vi "StopCalibration.vi"(7 "LVWSR":refnum<class "Web Request.lvclass">) -> ()   [LabVIEW 2014]
uses:
  <vilib>/wsapi/Web Request.lvclass
  Controller/Messages/Send Stop Calibration MSG/Send Stop Calibration MSG.lvclass
  Controller/Controller.lvclass
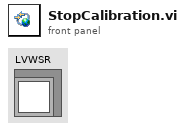
[diagram p1: front panel]
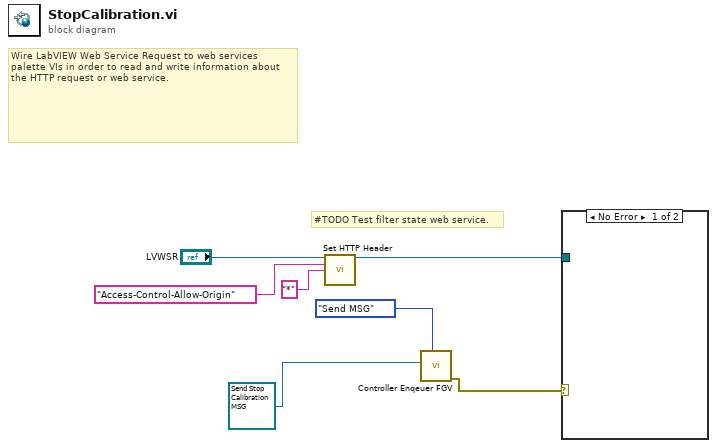
[diagram p0: block diagram]
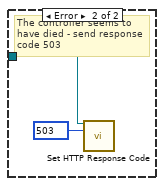
[diagram p2: hidden frame]
diagram:
  # "#TODO Test filter state web service."
  # "Wire LabVIEW Web Service Request to web services palette VIs in order to read and write information about the HTTP request or web service."
  n1 = call <vilib>:"Set HTTP Header.vi"("LabVIEW Web Service Request"="LVWSR", "header"="Access-Control-Allow-Origin", "header value"="*") -> ("LabVIEW Web Service Request out"=w5:refnum<class "Web Request.lvclass">)  [unwired: 11 in, 1 out]
  n2 = call "Controller Enqeuer FGV.vi"("State"=enum16{"Store", "Send MSG"}."Send MSG", "MSG"=refnum<class "Send Stop Calibration MSG.lvclass"> refnum ("Controller:Send Stop Calibration MSG.lvclass")) -> ("error out"=w1:errorcluster)  [unwired: 9 in]
  n3 = case shown="No Error" w1 {
    tunnel: w5 -> [_ w8]
    frame No Error {
    }
    frame Error {
      w9 = 503 items=["100"=100, "101"=101, "200"=200, "201"=201, "202"=202, "203"=203, "204"=204, "205"=205, "206"=206, "300"=300, "301"=301, "302"=302, "303"=303, "304"=304, "305"=305, "306"=306, "307"=307, "400"=400, "401"=401, "402"=402, "403"=403, "404"=404, "405"=405, "406"=406, "407"=407, "408"=408, "409"=409, "410"=410, "411"=411, "412"=412, "413"=413, "414"=414, "415"=415, "416"=416, "417"=417, "500"=500, "501"=501, "502"=502, "503"=503, "504"=504, "505"=505] ("response code (200)")
      # "The controller seems to have died - send response code 503"
      n4 = call <vilib>:"Set HTTP Response Code.vi"("LabVIEW Web Service Request"=w8, "response code (200)"=w9) -> ()  [unwired: 12 in, 2 out]
    }
  }
